vi "ABB Read Spreadsheet text.vi"(4 "delimiter (comma)":string=",", 6 "transpose (no:F)":bool, 7 "format (%s":string="%s", 8 "remove trailng empty strings":bool, 9 "start of read offset (chars.:0 )":i32, 10 "number of rows (all:-1)":i32=-1, 11 "file path (dialog if empty)":path) -> (0 "EOF?":bool, 1 "mark after read (chars.)":i32, 2 "first row":string[](array[string]), 3 "all rows":string[][](array[string]), 5 "new file path (Not A Path if cancelled)":path)   [LabVIEW 2017]
doc: "Reads a specified number of lines or rows from a numeric text file beginning at a specified character offset and converts the data to a 2D single-precision array of numbers. You can optionally transpose the array. The VI opens the file beforehand and closes it afterwards. You can use this VI to read spreadsheet file saved in text format that have columns separated with tab characters and rows terminated with EOL characters. See the note on the diagram if your file has other separators or terminators.\n\nfile path is the path name of the file. If file path is empty (default value) or is Not A Path, the VI displays a File dialog box from which you can select a file. Error 43 occurs if the user cancels the dialog. \n\nnumber of rows is the maximum number of rows or lines the VI reads. The default value is -1 rows, which means to read the entire file. For this VI, a row is a character string ending with a carriage return, line feed, or a carriage return followed by a line feed; a string ending at the EOF; or a string that has the maximum line length specified by the max characters per row input.\n\nstart of read offset is the position in the file, measured in characters (or bytes), at which the VI begins reading.\n\nmax characters per row is the maximum number of characters the VI reads before ending the search for the end of a row or line. The default is 0, which means that there is no limit to the number of characters the VI reads.\n\ntranspose? Set TRUE to transpose the data after converting it from a string. The default value is FALSE.\n\nformat specifies how to convert the characters to numbers; the default is %.3f. Refer to the discussion of format strings and the Spreadsheet String To Array function in Chapter 6, String Functions, of the LabVIEW Function Reference Manual.\n\nnew file path is the path of the file from which the VI read data. You can use this output to determine the path of a file that you open using dialog. new file path returns Not A Path if the user selects Cancel from the dialog box.\n\nall rows is the data read from the file in the form of a 2D array of single-precision numbers.\n\nfirst row is the first row of the all rows array in the form of a 1D array of single-precision numbers. You can use this output when you want to read one row into a 1D array.\n\nmark after read is the location of the file mark after the read; it points to the character in the file following the last character read.\n\nEOF? is TRUE if you attempt to read past the end of file."
panel:
  out "Array":i32[](array[numeric])
  in  "type (empty)":string[][](array[string])
  in  "max characters/row  (no limit:0)":i32
  # "row\ncolumn"
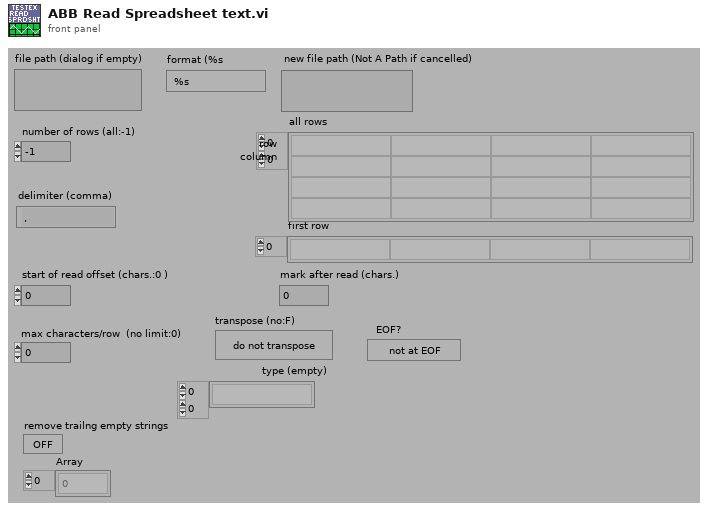
[diagram p1: front panel]
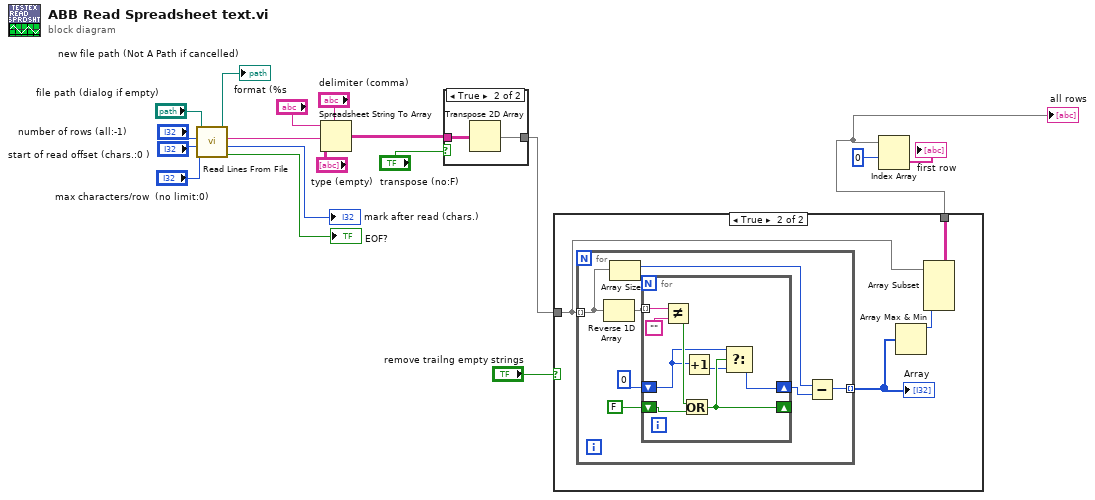
[diagram p0: block diagram]
diagram:
  n1 = call <vilib>:"Read Lines From File.vi"("file path (dialog if empty)"="file path (dialog if empty)", "number of lines (all:-1)"="number of rows (all:-1)", "start of read offset (chars.:0)"="start of read offset (chars.:0 )", "[max characters per line]  (no limit:0)"="max characters/row  (no limit:0)") -> ("new file path (Not A Path if cancelled)"=→"new file path (Not A Path if cancelled)":path, "line string"=w14:string, "mark after read (chars.)"=→"mark after read (chars.)":i32, "EOF?"=→"EOF?":bool)  [unwired: 2 in]
  n2 = Spreadsheet String To Array(delimiter (Tab)="delimiter (comma)", format string="format (%s", spreadsheet string=w14, array type (2D Dbl)="type (empty)") -> (array=w4:string[][])
  n3 = case shown="True" "transpose (no:F)" {
    tunnel: [w19 w21] -> w2
    tunnel: w4 -> [w19 w20]
    frame False {
    }
    frame True {
      n4 = Transpose 2D Array(2D array=w20) -> (transposed array=w21:string[][])
    }
  }
  n5 = case shown="True" "remove trailng empty strings" {
    tunnel: w2 -> [w22 w25]
    tunnel: [w22 w24] -> w1
    frame False {
    }
    frame True {
      n6 = for {
        tunnel: w25 -> [w33] mode=indexing
        tunnel: [w29] -> w26 mode=indexing
        n7 = Reverse 1D Array(array=w33) -> (reversed array=w31:string[])
        n8 = Array Size(array=w33) -> (size(s)=w28:i32)
        n9 = for {
          shift-right: [w34] -> w27
          shift-left: 0 -> [w35]
          shift-right: [w37] -> _
          shift-left: FALSE -> [w39]
          tunnel: w31 -> [w41] mode=indexing
          n10 = Not Equal?(x=w41, y="") -> (x != y?=w38:bool)
          n11 = Or(x=w38, y=w39) -> (x .or. y?=w37:bool)
          n12 = Increment(x=w35) -> (x+1=w36:i32)
          n13 = Select(t=w35, s=w37, f=w36) -> (s? t:f=w34:i32)
        }
        n14 = Subtract(x=w28, y=w27) -> (x-y=w29:i32)
      }
      "Array" <- w26
      n15 = Array Max & Min(array=w26) -> (max value=w23:i32)  [unwired: 3 out]
      n16 = Array Subset(array=w25, length (col)=w23) -> (w24:string[][])  [unwired: 3 in]
    }
  }
  "all rows" <- w1
  n17 = Index Array(array=w1, index (row)=0) -> (element=→"first row":string[])  [unwired: 1 in]
